vi "Status Set Register.vi"(7 "Val":i32 format="%.0g", 8 "error in (no error)":errorcluster {"code" format="%.0x"}, 9 "SubRegister (Condition)":i32(ring) items=["Condition", "Negative Transition", "Positive Transition", "Event", "Enable"], 10 "Register (Status Byte)":i32(ring) items=["Status Byte", "Standard Event", "Operation", "Questionable", "Ques Limit"], 11 "instrument handle":refnum<k15>) -> (0 "error out":errorcluster {"code" format="%.0x"}, 3 "instrument handle out":refnum<k15>)   [LabVIEW 2014, in "Agilent NA.lvlib"]
doc: "Read and write instrument status registers. All Event and Condition registers and the Status byte are read only."
uses:
  Agilent NA.lvlib
  AgNA.dll
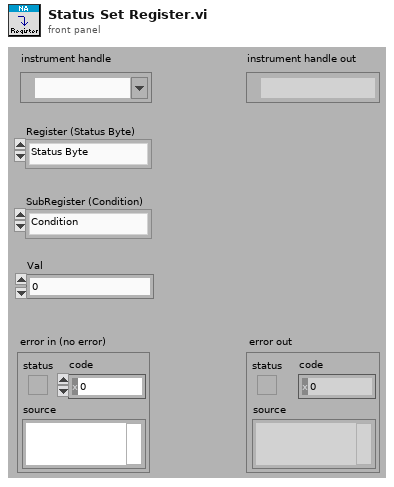
[diagram p1: front panel]
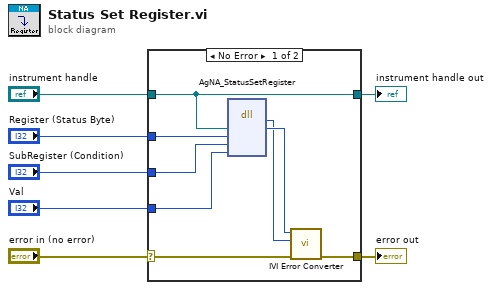
[diagram p0: block diagram]
diagram:
  n1 = case shown="No Error" "error in (no error)" {
    selector: "error in (no error)" -> [w13 w17]
    tunnel: [w12 w17] -> w7
    tunnel: "Register (Status Byte)" -> [w11 _]
    tunnel: "SubRegister (Condition)" -> [w10 _]
    tunnel: "Val" -> [w9 _]
    tunnel: [w8 w16] -> w2
    tunnel: "instrument handle" -> [w8 w16]
    frame No Error {
      n2 = dll-call lib="AgNA**.dll" fn="AgNA_StatusSetRegister"("Vi"=w8, "Register"=w11, "SubRegister"=w10, "Val"=w9) -> (w14:i32, "Vi"=w15:u32)  [unwired: 6 in, 2 out]
      n3 = call "IVI Error Converter.vi"("error in (no error)"=w13, "IVI error code (0)"=w14, "instrument handle"=w15) -> ("error out"=w12:errorcluster)  [unwired: 7 in, 1 out]
    }
    frame Error {
    }
  }
  "error out" <- w7
  "instrument handle out" <- w2
